vi "Drivetrain Loop_BASE_13624.vi"(9 "In 2":dbl, 11 "In 1":dbl) -> (1 "Out 2":dbl, 3 "Out 1":dbl)   [LabVIEW 2015]
uses:
  Robot Global Data.vi
  <vilib>/Rock Robotics/WPI/Solenoid/Deprecated/WPI_SolenoidSetBool.vi
  Common Code/Change Detect Boolean.vi
  Common Code/Drivetrain Modes.ctl
panel:
  in  "SavedTime1":dbl
  in  "SavedTime2":dbl
  out "Modes":T1=enum."Vision Targeting"
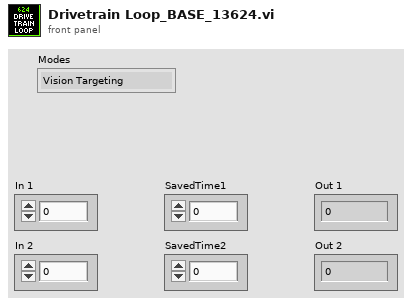
[diagram p1: front panel]
types:
  T1 = typedef "Drivetrain Modes.ctl" = enum16{"Climb", "Manual", "Vision Targeting", "PID Distance Drive", "Hybrid"}
  T2 = typedef "Drivetrain Commands.ctl" = cluster{"Y Power":dbl, "Turn Power":dbl, "1st Gear?":bool, "Modes":T1, "Heading Target":dbl, "X Max Speed":dbl, "Y Max Speed":dbl, "X Min Speed":dbl, "Y Min Speed":dbl, "Y Target":dbl}
  T3 = typedef "Dashboard Control Data.ctl" = cluster{"Auton Loops":dbl, "Shooter Presets":T4, "Encoder Control":T6, "Steer PID output":cluster{"output high":dbl, "output low":dbl}, " Steer PID gains":cluster{"proportional gain (Kc)":dbl, "integral time (Ti, min)":dbl, "derivative time (Td, min)":dbl}, "Drivetrain Settings":T7, "Vision Packet":T8, "Dashboard Drivetrain Command":T9, "Intake Command Cluster":T11}
  T4 = typedef "Shooter Presets.ctl" = cluster{"Batter Shot":T5, "Low Bar Curve Shot":T5, "Deep Middle Shot":T5, "Manual Shot":T5, "Left Ticks Per Rotation":dbl, "Right Ticks Per Rotation":dbl, "Low Bar Shot":T5, "Shooter RPM Tolerance":dbl, "IIR Filter Power":dbl, "Trigger Power":dbl, "Fire from Load Delay":i32, "Angle Pot Scale Factor":dbl, "Angle Pot Zero":dbl, "Shooter Deck Length":dbl, "String Pot Dist From Pivot":dbl, "Angle PID gains":cluster{"proportional gain (Kc)":dbl, "integral time (Ti, min)":dbl, "derivative time (Td, min)":dbl}, "Angle Motor Output Range":cluster{"output high":dbl, "output low":dbl}, "Shooter Angle Tolerance":dbl}
  T5 = typedef "Shot Presets.ctl" = cluster{"Left Wheel RPM":dbl, "Right Wheel RPM":dbl, "Angle":dbl}
  T6 = typedef "Encoder Control.ctl" = cluster{"Right Tick Constat":dbl, "Left Tick Constant":dbl, "Reset?":bool, "Y Dist":cluster{"PID gains":cluster{"proportional gain (Kc)":dbl, "integral time (Ti, min)":dbl, "derivative time (Td, min)":dbl}}, "Y Stop Thresh":dbl, "Y Stop Speed":dbl}
  T7 = typedef "Drivetrain Settings.ctl" = cluster{"Gyro Tolerance":dbl, "Throttle Ramp (ms)":dbl, "Angular rate compensation":bool, "Throttle to Rate Scale":dbl, "Rate compensation gain":dbl}
  T8 = typedef "Vision Packet.ctl" = cluster{"Distance":dbl, "Center X":dbl, "Center Y":dbl, "Found Target?":bool}
  T9 = typedef "Dashboard Drivetrain Command.ctl" = cluster{"Drivetrain Vision":T10, "Vision Scale Down Speed":dbl, "Vision PID gains":cluster{"proportional gain (Kc)":dbl, "integral time (Ti, min)":dbl, "derivative time (Td, min)":dbl}}
  T10 = typedef "Drivetrain Vision.ctl" = cluster{"High parameters":dbl, "Low parameters":dbl}
  T11 = typedef "Intake Command Cluster.ctl" = cluster{"Intake Speed":dbl, "Turn In Speed":dbl, "Turn Out Speed":dbl, "HP Load Speed":dbl, "Unload Speed":dbl, "Right Pot 0":dbl, "Left Pot 0":dbl, "Trigger Power":dbl}
  T12 = typedef "WPI_SolenoidDevRef.ctl" = cluster{"DevStatus":errorcluster, "Pneumatics Control Module":u8, "Forward Solenoid Channel":T13, "Reverse Solenoid Channel":T13}
  T13 = typedef "WPI_SolenoidChannel.ctl" = enum8{"Solenoid 0", "Solenoid 1", "Solenoid 2", "Solenoid 3", "Solenoid 4", "Solenoid 5", "Solenoid 6", "Solenoid 7", "Invalid"}
  T14 = typedef "Dist Drive Status.ctl" = cluster{"Y In Range":bool, "X In Range":bool, "Gyro In Range":bool, "Y Dist":dbl, "X Dist":dbl, "Gyro":dbl}
  T15 = typedef "Drivetrain Status Cluster.ctl" = cluster{"Modes":T1, "Y (Throttle)":dbl, "X (Steer)":dbl, "Gyro In Range?":bool, "Distance Drive Finished?":bool, "Stop Eject Lockout":bool, "Dist Drive Status":T14, "Y Target":dbl, "Heading Target":dbl, "Vision Target Aligned?":bool, "Gear":dbl, "1st Gear Time":dbl, "2nd Gear Time":dbl, "Gyro Angle":dbl}
  T16 = typedef "WPI_MotorControlDeviceRef.ctl" = cluster{"DeviceStatus":errorcluster, "Type":T17, "PWM":cluster{"PWM Channel":T18, "DeadBand":T19}, "CAN":cluster{"Device Number":u8, "Control Mode":T20, "Semaphore":T21, "Max Vout":dbl, "TalonSRX Control Mode":T22}, "Invert":bool}
  T17 = typedef "WPI_MotorControlType.ctl" = enum16{"PWM", "CAN", "CANTalonSRX"}
  T18 = typedef "FPGA_DIOPWMChannel.ctl" = enum8{"PWM 0", "PWM 1", "PWM 2", "PWM 3", "PWM 4", "PWM 5", "PWM 6", "PWM 7", "PWM 8", "PWM 9", "PWM MXP 0", "PWM MXP 1", "PWM MXP 2", "PWM MXP 3", "PWM MXP 4", "PWM MXP 5", "PWM MXP 6", "PWM MXP 7", "PWM MXP 8", "PWM MXP 9", "Invalid"}
  T19 = typedef "WPI_PWMDeadband.ctl" = cluster{"Name":string, "maxPositivePwm":i32, "minPositivePwm":i32, "centerPwm":i32, "maxNegativePwm":i32, "minNegativePwm":i32, "angularRange":u16}
  T20 = typedef "WPI_CANJaguar_ControlMode.ctl" = enum8{"Percent VBus", "Current", "Speed", "Position", "Voltage"}
  T21 = typedef "Semaphore RefNum" = refnum<k1>
  T22 = typedef "WPI_CANTalonSRX_APIControlMode.ctl" = enum8{"Percent VBus", "Speed", "Position", "Slave", "Unchanged / Invalid", "Voltage Compensation", "Current", "Motion Profile"}
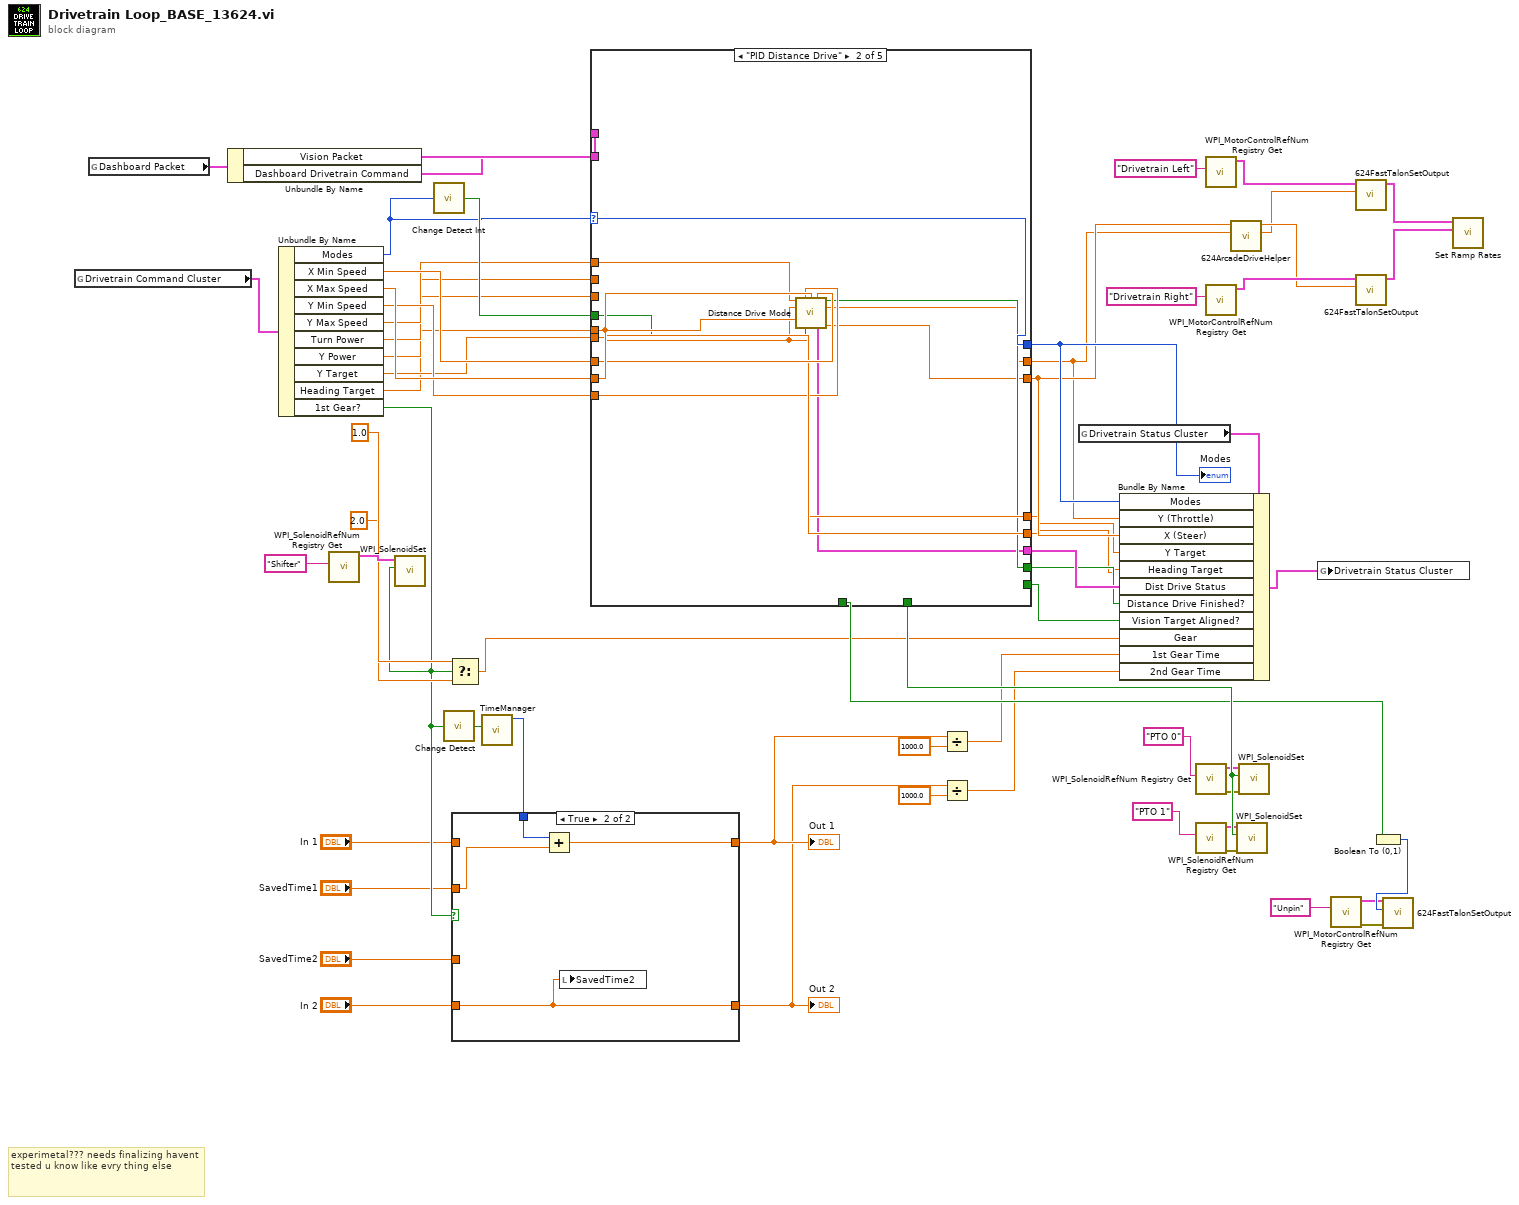
[diagram p0: block diagram]
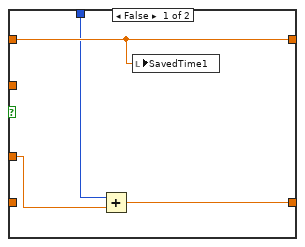
[diagram p2: hidden frame]
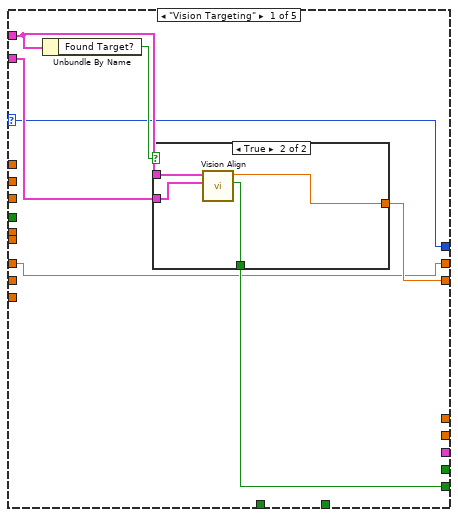
[diagram p3: hidden frame]
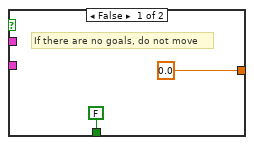
[diagram p4: hidden frame]
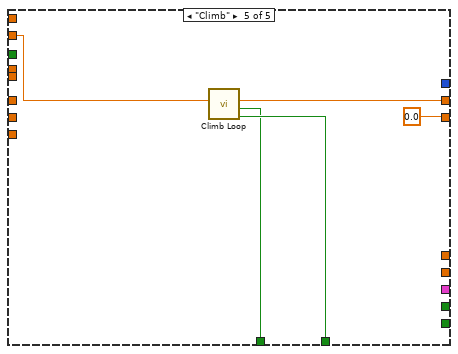
[diagram p7: hidden frame]
diagram:
  # "experimetal??? needs finalizing havent tested u know like evry thing else"
  n1 = global read "Robot Global Data.vi" "Drivetrain Command Cluster"() -> (w39:T2)
  n2 = global read "Robot Global Data.vi" "Dashboard Packet"() -> (w34:T3)
  n3 = Unbundle By Name(w34) -> ("Vision Packet"=w36:T8, "Dashboard Drivetrain Command"=w35:T9)
  n4 = Unbundle By Name(w39) -> ("Modes"=w48:T1, "X Min Speed"=w47:dbl, "X Max Speed"=w46:dbl, "Y Min Speed"=w45:dbl, "Y Max Speed"=w44:dbl, "Turn Power"=w43:dbl, "Y Power"=w42:dbl, "Y Target"=w41:dbl, "Heading Target"=w40:dbl, "1st Gear?"=w12:bool)
  n5 = call <vilib>:"WPI_SolenoidRefNum Registry Get.vi"("refnum name"="Shifter") -> ("SolenoidDevRef"=w61:T12)  [unwired: 9 in, 1 out]
  n6 = call-poly <vilib>:"WPI_SolenoidSet.vi"("Value"=w12, "SolenoidDevRef"=w61) -> ()  [unwired: 8 in, 2 out]
  n7 = call "Change Detect Int.vi"("In"=w48) -> ("Changed?"=w57:bool)
  n8 = call-poly "Change Detect.vi"("In"=w12) -> ("Changed?"=w13:bool)
  n9 = Select(t=1.0, s=w12, f=2.0) -> (s? t:f=w15:dbl)
  n10 = call "TimeManager.vi"("Reset?"=w13) -> ("Time Since Reset"=w7:u32)  [unwired: 9 in, 1 out]
  n11 = case shown="True" w12 {
    tunnel: "SavedTime1" -> [_ w69]
    tunnel: "SavedTime2" -> [w65 _]
    tunnel: "In 1" -> [w66 _]
    tunnel: "In 2" -> [_ w70]
    tunnel: [w63 w70] -> w2
    tunnel: [w66 w67] -> w3
    tunnel: w7 -> [w64 w68]
    frame False {
      n12 = Add(x=w64, y=w65) -> (x+y=w63:dbl)
      n13 = local write "SavedTime1"(w66) -> ()
    }
    frame True {
      n14 = Add(x=w68, y=w69) -> (x+y=w67:dbl)
      n15 = local write "SavedTime2"(w70) -> ()
    }
  }
  "Out 1" <- w3
  "Out 2" <- w2
  n16 = case shown="\"PID Distance Drive\"" w48 {
    selector: w48 -> [w72 w95 _ w98 _]
    tunnel: w47 -> [w71 w92 _ _ _]
    tunnel: w46 -> [_ w94 _ _ _]
    tunnel: w45 -> [_ w90 _ _ _]
    tunnel: [w71 w87 _ w97 w101] -> w51
    tunnel: [w76 w85 _ w96 0.0] -> w52
    tunnel: [w72 w95 _ w98 _] -> w60
    tunnel: w57 -> [_ w84 _ _ _]
    tunnel: [w77 _ _ _ _] -> w20
    tunnel: [_ w88 _ _ _] -> w18
    tunnel: [_ w86 _ _ _] -> w19
    tunnel: [_ w89 _ _ _] -> w16
    tunnel: [_ w91 _ _ _] -> w17
    tunnel: w42 -> [_ _ _ w97 w100]
    tunnel: w44 -> [_ w93 _ _ _]
    tunnel: w40 -> [_ w91 _ _ _]
    tunnel: w43 -> [_ _ _ w96 _]
    tunnel: w41 -> [_ w89 _ _ _]
    tunnel: w36 -> [w75 _ _ _ _]
    tunnel: w35 -> [w73 _ _ _ _]
    tunnel: [_ _ _ _ w103] -> w33
    tunnel: [_ _ _ _ w102] -> w26
    frame "Vision Targeting" {
      n17 = Unbundle By Name(w75) -> ("Found Target?"=w74:bool)
      n18 = case shown="True" w74 {
        tunnel: [0.0 ("Turn Power") w82] -> w76
        tunnel: w73 -> [_ w80]
        tunnel: w75 -> [_ w81]
        tunnel: [FALSE ("Aligned?") w83] -> w77
        frame False {
          # "If there are no goals, do not move"
        }
        frame True {
          n19 = call "Vision Align.vi"("Dashboard Drivetrain Command"=w80, "Vision Packet"=w81) -> ("Aligned?"=w83:bool, "Turn Power"=w82:dbl)  [unwired: 8 in]
        }
      }
    }
    frame "PID Distance Drive" {
      n20 = call "Distance Drive Mode.vi"("Y Output High"=w93, "Y Output Low"=w90, "X Output High"=w94, "X Output Low"=w92, "Y target"=w89, "Heading target"=w91, "Reinitialize"=w84) -> ("isFinished"=w88:bool, "Y out"=w87:dbl, "Dist Drive Status"=w86:T14, "X out"=w85:dbl)  [unwired: 5 in]
    }
    frame "Hybrid" {
    }
    frame "Manual", Default {
    }
    frame "Climb" {
      n21 = call "Climb Loop.vi"("Y Power"=w100) -> ("Engage"=w103:bool, "Unpin"=w102:bool, "Y Power Output"=w101:dbl)  [unwired: 8 in]
    }
  }
  "Modes" <- w60
  n22 = Divide(x=w3, y=1000.0) -> (x/y=w5:dbl)
  n23 = Divide(x=w2, y=1000.0) -> (x/y=w1:dbl)
  n24 = global read "Robot Global Data.vi" "Drivetrain Status Cluster"() -> (w14:T15)
  n25 = Bundle By Name(cluster=w14, "Modes"=w60, "Y (Throttle)"=w51, "X (Steer)"=w52, "Y Target"=w16, "Heading Target"=w17, "Dist Drive Status"=w19, "Distance Drive Finished?"=w18, "Vision Target Aligned?"=w20, "Gear"=w15, "1st Gear Time"=w5, "2nd Gear Time"=w1) -> (w21:T15)
  n26 = call <vilib>:"WPI_SolenoidRefNum Registry Get.vi"("refnum name"="PTO 0") -> ("error out"=w29:errorcluster, "SolenoidDevRef"=w28:T12)  [unwired: 9 in]
  n27 = call <vilib>:"WPI_SolenoidRefNum Registry Get.vi"("refnum name"="PTO 1") -> ("error out"=w32:errorcluster, "SolenoidDevRef"=w31:T12)  [unwired: 9 in]
  n28 = call <vilib>:"WPI_MotorControlRefNum Registry Get.vi"("refnum name"="Drivetrain Left") -> ("MotorControlDevRef"=w55:T16)  [unwired: 9 in, 1 out]
  n29 = call <vilib>:"WPI_MotorControlRefNum Registry Get.vi"("refnum name"="Drivetrain Right") -> ("MotorControlDevRef"=w56:T16)  [unwired: 9 in, 1 out]
  n30 = call "624ArcadeDriveHelper.vi"("Y Power"=w51, "Turn Power"=w52) -> ("Left"=w49:dbl, "Right"=w50:dbl)  [unwired: 8 in]
  n31 = call-poly <vilib>:"WPI_SolenoidSet.vi"("error in (no error)"=w32, "Value"=w33, "SolenoidDevRef"=w31) -> ()  [unwired: 7 in, 2 out]
  n32 = call-poly <vilib>:"WPI_SolenoidSet.vi"("error in (no error)"=w29, "Value"=w33, "SolenoidDevRef"=w28) -> ()  [unwired: 7 in, 2 out]
  n33 = global write "Robot Global Data.vi" "Drivetrain Status Cluster"(w21) -> ()
  n34 = call <vilib>:"WPI_MotorControlRefNum Registry Get.vi"("refnum name"="Unpin") -> ("error out"=w24:errorcluster, "MotorControlDevRef"=w23:T16)  [unwired: 9 in]
  n35 = call "624FastTalonSetOutput.vi"("Output"=w49, "MotorControlDevRef"=w55) -> ("MotorControlDevRef"=w54:T16)  [unwired: 8 in, 1 out]
  n36 = call "624FastTalonSetOutput.vi"("Output"=w50, "MotorControlDevRef"=w56) -> ("MotorControlDevRef"=w53:T16)  [unwired: 8 in, 1 out]
  n37 = Boolean To (0,1)(Boolean=w26) -> (0, 1=w25:i16)
  n38 = call "624FastTalonSetOutput.vi"("error in (no error)"=w24, "Output"=w25, "MotorControlDevRef"=w23) -> ()  [unwired: 7 in, 2 out]
  n39 = call "Set Ramp Rates.vi"("DT Right"=w53, "DT Left"=w54) -> ()  [unwired: 10 in]
